vi "Find Background Image.vi"(10 "Backgroundic Qualities":T1(array[cluster]), 11 "Images":refnum<class "SVGImage.lvclass">[](array[class])) -> (2 "Backgroundic Qualities":T2, 3 "Background Image":refnum<class "SVGImage.lvclass">, 5 "index of element":i32)   [LabVIEW 2019, in "SVGImage.lvclass"]
uses:
  SVGImage.lvclass
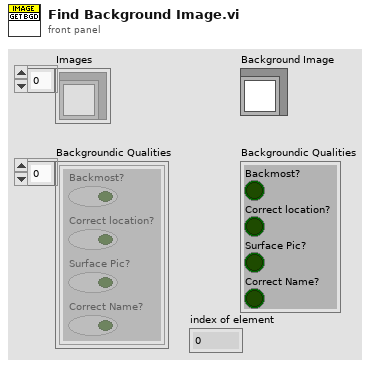
[diagram p1: front panel]
types:
  T1 = cluster{"Backmost?":bool, "Correct location?":bool, "Surface Pic?":bool, "Correct Name?":bool}[]
  T2 = cluster{"Backmost?":bool, "Correct location?":bool, "Surface Pic?":bool, "Correct Name?":bool}
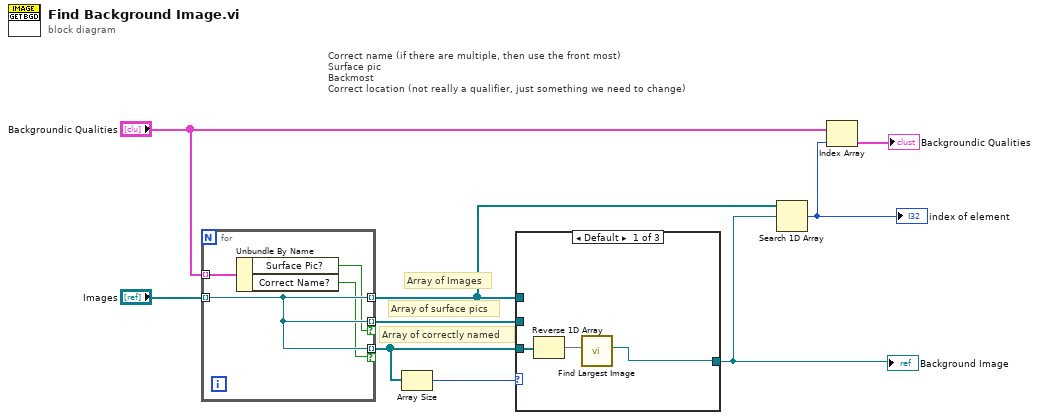
[diagram p0: block diagram]
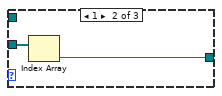
[diagram p2: hidden frame]
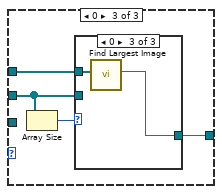
[diagram p3: hidden frame]
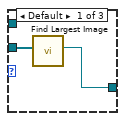
[diagram p4: hidden frame]
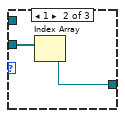
[diagram p5: hidden frame]
diagram:
  # "Array of correctly named"
  # "Array of surface pics"
  # "Array of Images"
  # "Correct name (if there are multiple, then use the front most)\nSurface pic\nBackmost\nCorrect location (not really a qualifier, just something we need to change)"
  n1 = for {
    tunnel: "Backgroundic Qualities" -> [w13] mode=indexing
    tunnel: "Images" -> [w12] mode=indexing
    tunnel: [w12] -> w6 mode=indexing
    tunnel: [w12] -> w7 mode=indexing if=w10
    tunnel: [w12] -> w8 mode=indexing if=w11
    n2 = Unbundle By Name(w13) -> ("Surface Pic?"=w10:bool, "Correct Name?"=w11:bool)
  }
  n3 = Array Size(array=w8) -> (size(s)=w9:i32)
  n4 = case shown="Default" w9 {
    tunnel: w8 -> [w16 w18 _]
    tunnel: [w14 w17 w20] -> w5
    tunnel: w7 -> [_ _ w19]
    tunnel: w6 -> [_ _ w21]
    frame Default {
      n5 = Reverse 1D Array(array=w16) -> (reversed array=w15:refnum<class "SVGImage.lvclass">[])
      n6 = call "Find Largest Image.vi"("Images"=w15) -> ("Largest Image"=w14:refnum<class "SVGImage.lvclass">)  [unwired: 10 in]
    }
    frame 1 {
      n7 = Index Array(array=w18) -> (element=w17:refnum<class "SVGImage.lvclass">)  [unwired: 1 in]
    }
    frame 0 {
      n8 = Array Size(array=w19) -> (size(s)=w22:i32)
      n9 = case shown="0" w22 {
        tunnel: w21 -> [_ _ w28]
        tunnel: [w23 w25 w27] -> w20
        tunnel: w19 -> [w24 w26 _]
        frame Default {
          n10 = call "Find Largest Image.vi"("Images"=w24) -> ("Largest Image"=w23:refnum<class "SVGImage.lvclass">)  [unwired: 10 in]
        }
        frame 1 {
          n11 = Index Array(array=w26) -> (element=w25:refnum<class "SVGImage.lvclass">)  [unwired: 1 in]
        }
        frame 0 {
          n12 = call "Find Largest Image.vi"("Images"=w28) -> ("Largest Image"=w27:refnum<class "SVGImage.lvclass">)  [unwired: 10 in]
        }
      }
    }
  }
  "Background Image" <- w5
  n13 = Search 1D Array(1D array=w6, element=w5) -> (index of element=w4:i32)  [unwired: 1 in]
  "index of element" <- w4
  n14 = Index Array(array="Backgroundic Qualities", index=w4) -> (element=→"Backgroundic Qualities":T2)
